vi "3_RGT_Worksheets.vi"   [LabVIEW 2014]
uses:
  <vilib>/Utility/NIReport.llb/NI_report.lvclass
  <vilib>/Utility/NIReport.llb/Excel/NI_Excel.lvclass
  <vilib>/Utility/NIReport.llb/Append Numeric Table to Report (wrap).vi
types:
  T1 = enum16{"Standard Report", "HTML", "Word", "Excel"}
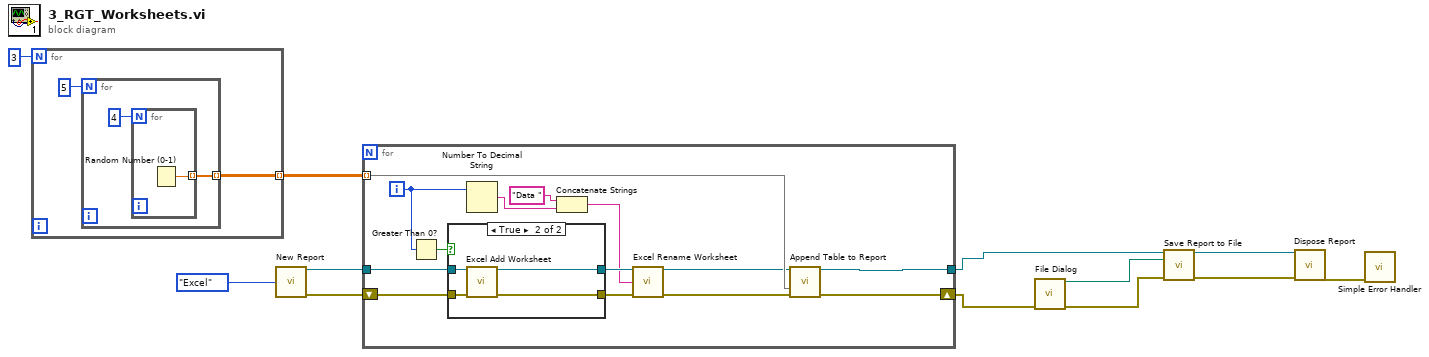
[diagram p0: block diagram]
diagram:
  n1 = for {
    N: 3 -> [_]
    tunnel: [w13] -> w8 mode=indexing
    n2 = for {
      N: 5 -> [_]
      tunnel: [w16] -> w13 mode=indexing
      n3 = for {
        N: 4 -> [_]
        tunnel: [w17] -> w16 mode=indexing
        n4 = Random Number (0-1)() -> (number: 0 to 1=w17:dbl)
      }
    }
  }
  n5 = call <vilib>:"New Report.vi"("report type"=T1."Excel") -> ("report out"=w10:refnum<class "NI_report.lvclass">, "error out"=w9:errorcluster)  [unwired: 13 in]
  n6 = for {
    tunnel: w8 -> [w20] mode=indexing
    shift-right: [w21] -> w3
    shift-left: w9 -> [w29]
    tunnel: w10 -> [w30]
    tunnel: [w18] -> w4
    i -> [w25]
    n7 = Greater Than 0?(x=w25) -> (x > 0?=w31:bool)
    n8 = case shown="True" w31 {
      tunnel: w30 -> [w33 w37]
      tunnel: w29 -> [w32 w36]
      tunnel: [w33 w35] -> w28
      tunnel: [w32 w34] -> w27
      frame False {
      }
      frame True {
        n9 = call <vilib>:"Excel Add Worksheet.vi"("report in"=w37, "error in (no error)"=w36) -> ("report out"=w35:refnum<class "NI_report.lvclass">, "error out"=w34:errorcluster)  [unwired: 12 in]
      }
    }
    n10 = Number To Decimal String(number=w25) -> (decimal integer string=w24:string)  [unwired: 1 in]
    n11 = Concatenate Strings("Data ", w24) -> (w23:string)
    n12 = call <vilib>:"Excel Rename Worksheet.vi"("report in"=w28, "worksheet name (\"\")"=w23, "error in (no error)"=w27) -> ("report out"=w19:refnum<class "NI_report.lvclass">, "error out"=w22:errorcluster)  [unwired: 11 in]
    n13 = call-poly <vilib>:"Append Table to Report.vi"("report in"=w19, "numerical data"=w20, "error in (no error)"=w22) -> ("report out"=w18:refnum<class "NI_report.lvclass">, "error out"=w21:errorcluster)  [unwired: 9 in, 2 out]
  }
  n14 = call "File Dialog"("error in"=w3) -> ("selected path"=w6:path, "error out"=w5:errorcluster)  [unwired: 11 in, 2 out]
  n15 = call-dynamic "Save Report to File.vi"("report in"=w4, "report file path"=w6, "error in (no error)"=w5) -> ("report out"=w2:refnum<class "NI_report.lvclass">, "error out"=w1:errorcluster)  [unwired: 11 in]
  n16 = call-dynamic "Dispose Report.vi"("report in"=w2, "error in (no error)"=w1) -> ("error out"=w7:errorcluster)  [unwired: 13 in]
  n17 = call <vilib>:"Simple Error Handler.vi"("error in (no error)"=w7) -> ()  [unwired: 4 in, 5 out]
